vi "create_z_intensity_tuples.vi"(8 "error in (no error)":errorcluster, 11 "TrajectoryAK101022Resonance in":refnum<class "TrajectoryAK101022Resonance.lvclass">) -> (0 "error out":errorcluster, 2 "z/intensity tuples":u32[](array[numeric]), 3 "TrajectoryAK101022Resonance out":refnum<class "TrajectoryAK101022Resonance.lvclass">)   [LabVIEW 2010, in "TrajectoryAK101022Resonance.lvclass"]
uses:
  TrajectoryAK101022Resonance.lvclass
  TrajectoryAK101022Resonance.lvclass/TrajectoryAK101022Resonance.ctl
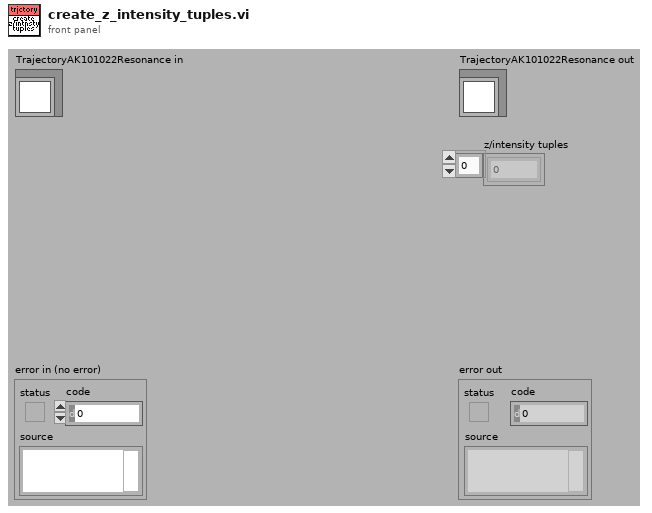
[diagram p1: front panel]
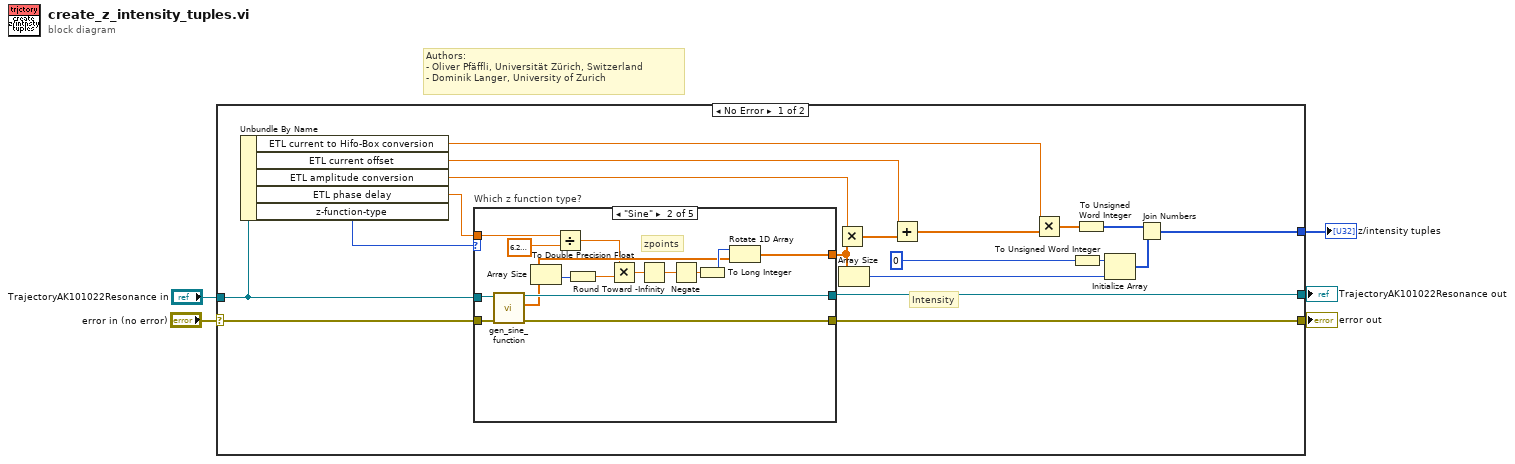
[diagram p0: block diagram]
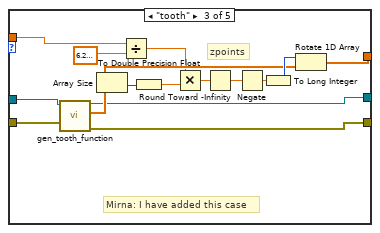
[diagram p3: hidden frame]
diagram:
  # "Authors: \n- Oliver Pfäffli, Universität Zürich, Switzerland\n- Dominik Langer, University of Zurich"
  n1 = case shown="No Error" "error in (no error)" {
    selector: "error in (no error)" -> [w16 w62]
    tunnel: [w12 w62] -> w4
    tunnel: [w11 w61] -> w2
    tunnel: "TrajectoryAK101022Resonance in" -> [w15 w61]
    tunnel: [w9 _] -> w1
    frame No Error {
      # "Intensity"
      n2 = Unbundle By Name(w15) -> ("ETL current to Hifo-Box conversion"=w23:dbl[unit], "ETL current offset"=w22:dbl[unit], "ETL amplitude conversion"=w24:dbl[unit], "ETL phase delay"=w13:dbl[unit], "z-function-type"=w14:enum16{"Sine", "tooth", "Stack", "Step"})
      n3 = case "Which z function type?" shown="\"Sine\"" w14 {
        tunnel: w16 -> [w25 w36 w46 w58 w60]
        tunnel: [w25 w35 w44 w58 w60] -> w12
        tunnel: w15 -> [w26 w34 w47 w57 w59]
        tunnel: [w26 w33 w45 w57 w59] -> w11
        tunnel: [_ w31 w42 _ _] -> w7
        tunnel: w13 -> [_ w29 w43 _ _]
        frame Default {
        }
        frame "Sine" {
          # "zpoints"
          n4 = call "gen_sine_function.vi"("error in (no error)"=w36, "TrajectoryAK101022Resonance in"=w34) -> ("error out"=w35:errorcluster, "z points"=w32:dbl[unit][], "TrajectoryAK101022Resonance out"=w33:refnum<class "TrajectoryAK101022Resonance.lvclass">)  [unwired: 6 in, 1 out]
          n5 = Array Size(array=w32) -> (size(s)=w40:i32)
          n6 = Divide(x=w29, y=dbl[unit] 6.283185307179586) -> (x/y=w28:dbl)
          n7 = To Double Precision Float(number=w40) -> (double precision float=w41:dbl)
          n8 = Multiply(x=w28, y=w41) -> (x*y=w27:dbl)
          n9 = Round Toward -Infinity(1:w27) -> (0:w38:dbl)
          n10 = Negate(x=w38) -> (-x=w37:dbl)
          n11 = To Long Integer(number=w37) -> (32bit integer=w39:i32)
          n12 = Rotate 1D Array(1:w32, 2:w39) -> (0:w31:dbl[unit][])
        }
        frame "tooth" {
          # "zpoints"
          # "Mirna: I have added this case"
          n13 = call "gen_tooth_function.vi"("error in (no error)"=w46, "TrajectoryAK101022Resonance in"=w47) -> ("error out"=w44:errorcluster, "z points"=w50:dbl[unit][], "TrajectoryAK101022Resonance out"=w45:refnum<class "TrajectoryAK101022Resonance.lvclass">)  [unwired: 6 in, 1 out]
          n14 = Array Size(array=w50) -> (size(s)=w54:i32)
          n15 = Divide(x=w43, y=dbl[unit] 6.283185307179586) -> (x/y=w48:dbl)
          n16 = To Double Precision Float(number=w54) -> (double precision float=w55:dbl)
          n17 = Multiply(x=w48, y=w55) -> (x*y=w56:dbl)
          n18 = Round Toward -Infinity(1:w56) -> (0:w52:dbl)
          n19 = Negate(x=w52) -> (-x=w51:dbl)
          n20 = To Long Integer(number=w51) -> (32bit integer=w53:i32)
          n21 = Rotate 1D Array(1:w50, 2:w53) -> (0:w42:dbl[unit][])
        }
        frame "Stack" {
        }
        frame "Step" {
        }
      }
      n22 = Multiply(x=w24, y=w7) -> (x*y=w18:dbl[unit][])
      n23 = Array Size(array=w7) -> (size(s)=w6:i32)
      n24 = Add(x=w22, y=w18) -> (x+y=w17:dbl[unit][])
      n25 = Multiply(x=w23, y=w17) -> (x*y=w20:dbl[])
      n26 = To Unsigned Word Integer(number=u16 0 ("index")) -> (unsigned 16bit integer=w10:u16)
      n27 = To Unsigned Word Integer(number=w20) -> (unsigned 16bit integer=w19:u16[])
      n28 = Initialize Array(w10, w6) -> (w8:u16[])
      n29 = Join Numbers(hi=w19, lo=w8) -> ((hi.lo)=w9:u32[])
    }
    frame Error {
    }
  }
  "error out" <- w4
  "TrajectoryAK101022Resonance out" <- w2
  "z/intensity tuples" <- w1
